vi "Open Debug Window.vi"(8 "error in (no error)":errorcluster) -> (0 "error out":errorcluster)   [LabVIEW 2020, in "Tamer.lvlib" / "Tamer.lvclass"]
uses:
  Tamer.lvclass
  Debug Info Display.vi
panel:
  # "TAMER::Debug Window"
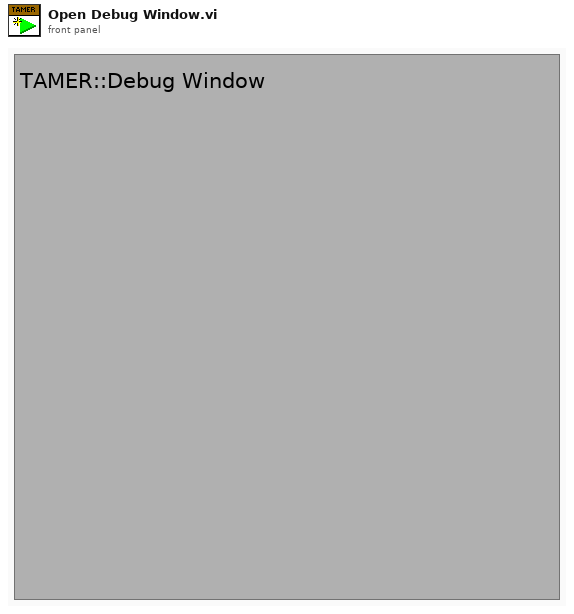
[diagram p1: front panel]
types:
  T1 = enum32{"Invalid", "Standard", "Closed", "Hidden", "Minimized", "Maximized"}
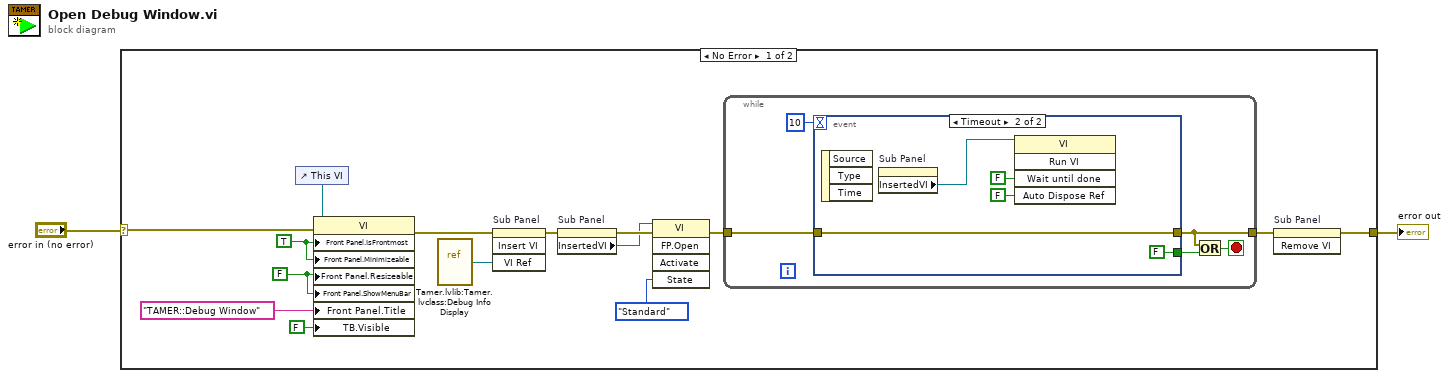
[diagram p0: block diagram]
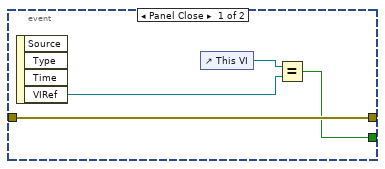
[diagram p2: hidden frame]
diagram:
  n1 = case shown="No Error" "error in (no error)" {
    selector: "error in (no error)" -> [w9 w32]
    tunnel: [w3 w32] -> w1
    frame No Error {
      w7 = FALSE ("Front Panel Window:Resizable")
      w8 = TRUE ("Front Panel Window:Is Frontmost")
      n2 = control-ref of="This VI"() -> (w11:refnum<vi>)
      n3 = property class="VI"(reference=w11, error in=w9, "Front Panel.IsFrontmost"=w8, "Front Panel.Minimizeable"=w8, "Front Panel.Resizeable"=w7, "Front Panel.ShowMenuBar"=w7, "Front Panel.Title"="TAMER::Debug Window" ("Front Panel Window:Title"), "TB.Visible"=FALSE ("Tool Bar:Visible")) -> (error out=w10:errorcluster)  [unwired: 1 out]
      n4 = vi-ref "Tamer.lvlib:Tamer.lvclass:Debug Info Display.vi"() -> (w12:refnum<vi>)
      n5 = invoke on="Sub Panel" class="SubPnl" method="Insert VI"(error in=w10, "VI Ref"=w12) -> (error out=w16:errorcluster)  [unwired: 2 in, 3 out]
      n6 = property on="Sub Panel" class="SubPnl"(error in=w16) -> (error out=w15:errorcluster, "InsertedVI"=w14:refnum<vi>)  [unwired: 1 in, 1 out]
      n7 = invoke class="VI" method="FP.Open"(reference=w14, error in=w15, "State"=T1."Standard") -> (error out=w13:errorcluster)  [unwired: 2 in, 4 out]
      n8 = while {
        tunnel: [w19] -> w4
        tunnel: w13 -> [w21]
        stop <- w20 stop-if-true
        n9 = event shown="[1] Timeout" {
          selector: _ -> [_ _]
          dyn-events: _ -> [_ _]
          timeout: 10 -> [_ _]
          tunnel: [w23 FALSE] -> w22
          tunnel: [w26 w28] -> w19
          tunnel: w21 -> [w26 w28]
          event Panel Close {
            n10 = event-data() -> ("VIRef"=w25:refnum<vi>)  [unwired: 1 in, 3 out]
            n11 = control-ref of="This VI"() -> (w24:refnum<vi>)
            n12 = Equal?(x=w24, y=w25) -> (x = y?=w23:bool)
          }
          event Timeout {
            n13 = event-data() -> ()  [unwired: 1 in, 3 out]
            n14 = property on="Sub Panel" class="SubPnl"() -> ("InsertedVI"=w31:refnum<vi>)  [unwired: 2 in, 2 out]
            n15 = invoke class="VI" method="Run VI"(reference=w31, "Wait until done"=FALSE ("Wait Until Done"), "Auto Dispose Ref"=FALSE ("Auto Dispose Reference")) -> ()  [unwired: 2 in, 5 out]
          }
        }
        n16 = Or(x=w19, y=w22) -> (x .or. y?=w20:bool)
      }
      n17 = invoke on="Sub Panel" class="SubPnl" method="Remove VI"(error in=w4) -> (error out=w3:errorcluster)  [unwired: 2 in, 2 out]
    }
    frame Error {
    }
  }
  "error out" <- w1
